vi "Graphics-Draw Reference Points.vi"(0 "XYGraph in":refnum<vi>, 7 "X values":dbl[](array[numeric]), 9 "Y values":dbl[](array[numeric])) -> ()   [LabVIEW 2015]
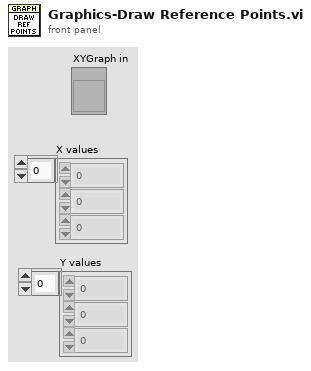
[diagram p1: front panel]
types:
  T1 = typedef "LVRectTypeDef.ctl" = cluster{"Left":i16, "Top":i16, "Right":i16, "Bottom":i16}
  T2 = cluster{"Width":u16, "Style":enum32{"Solid", "Dash", "Dot", "DashDot", "DashDotDot"}}
  T3 = typedef "LVPoint32TypeDef.ctl" = cluster{"Horizontal":i32, "Vertical":i32}
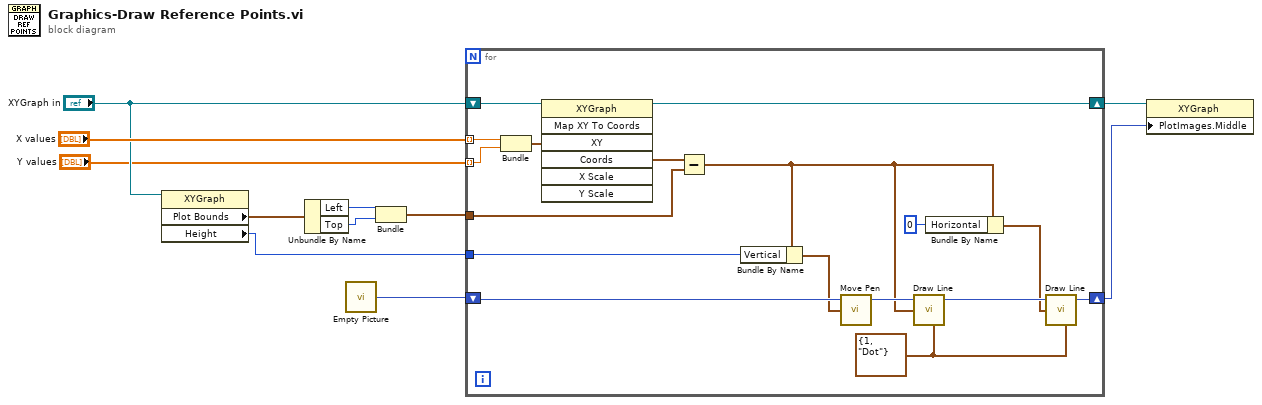
[diagram p0: block diagram]
diagram:
  n1 = property class="XYGraph"(reference="XYGraph in") -> ("Plot Bounds"=w6:T1, "Height"=w1:u32)  [unwired: 1 in, 2 out]
  n2 = Unbundle By Name(w6) -> ("Left"=w4:i16, "Top"=w3:i16)
  n3 = call "Empty Picture"() -> ("empty picture"=w11:picture)
  n4 = Bundle("Left"=w4, "Top"=w3) -> (w2:cluster{"Left":i16, "Top":i16})  [unwired: 1 in]
  n5 = for {
    tunnel: "X values" -> [w23] mode=indexing
    shift-right: [w18] -> w10
    shift-left: w11 -> [w28]
    shift-right: [w24] -> w9
    shift-left: "XYGraph in" -> [w27]
    tunnel: w2 -> [w22]
    tunnel: "Y values" -> [w20] mode=indexing
    tunnel: w1 -> [w15]
    w17 = T2 {"Width"=1, "Style"=enum."Dot"} ("pen")
    n6 = Bundle("Numeric"=w23, "Numeric"=w20) -> (w26:cluster{"Numeric":dbl, "Numeric":dbl})  [unwired: 1 in]
    n7 = invoke class="XYGraph" method="Map XY To Coords"(reference=w27, "XY"=w26) -> (reference out=w24:refnum<vi>, "Coords"=w16:T3)  [unwired: 5 in, 5 out]
    n8 = Subtract(x=w16, y=w22) -> (x-y=w14:T3)
    n9 = Bundle By Name(cluster=w14, "Vertical"=w15) -> (w21:T3)
    n10 = call <vilib>:"Move Pen.vi"("new position"=w21, "picture"=w28) -> ("new picture"=w25:picture)  [unwired: 3 in]
    n11 = call <vilib>:"Draw Line.vi"("picture"=w25, "end point"=w14, "pen"=w17) -> ("new picture"=w19:picture)  [unwired: 6 in]
    n12 = Bundle By Name(cluster=w14, "Horizontal"=0) -> (w12:T3)
    n13 = call <vilib>:"Draw Line.vi"("picture"=w19, "end point"=w12, "pen"=w17) -> ("new picture"=w18:picture)  [unwired: 6 in]
  }
  n14 = property class="XYGraph"(reference=w9, "PlotImages.Middle"=w10) -> ()  [unwired: 1 in, 2 out]
